vi "ENUM_Parse.vi"(8 "error":errorcluster, 9 "Secondary seporator(,)":string=",", 10 "Primary seperator(;)":string=";", 11 "Enum":variant) -> (0 "error out":errorcluster, 1 "Post Seperator array":string[](array[string]), 3 "Post Seperator":string, 5 "Name":string)   [LabVIEW 2015]
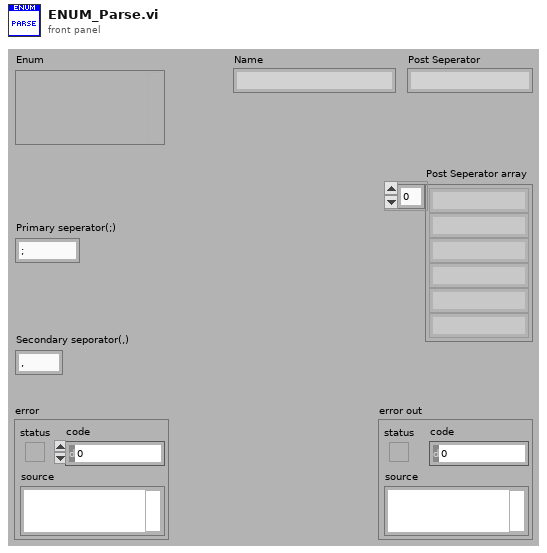
[diagram p1: front panel]
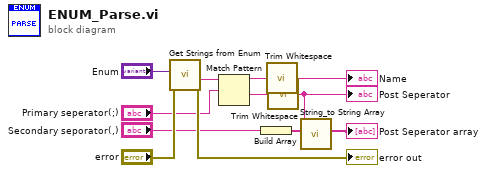
[diagram p0: block diagram]
diagram:
  n1 = call "Get Strings from Enum.vi"("error in (no error)"="error", "Enum"="Enum") -> ("error out"=→"error out":errorcluster, "String Value"=w1:string)  [unwired: 6 in, 2 out]
  n2 = Match Pattern(string=w1, regular expression="Primary seperator(;)") -> (before substring=w8:string, after substring=w6:string)  [unwired: 1 in, 2 out]
  n3 = Build Array("Secondary seporator(,)") -> (w3:string[])
  n4 = call <vilib>:"Trim Whitespace.vi"("string"=w8) -> ("trimmed string"=→"Name":string)  [unwired: 1 in]
  n5 = call <vilib>:"Trim Whitespace.vi"("string"=w6) -> ("trimmed string"=w5:string)  [unwired: 1 in]
  "Post Seperator" <- w5
  n6 = call "String_to String Array.vi"("Seperators (;)"=w3, "Input String"=w5) -> ("String Array Out Blanks Removed Out"=→"Post Seperator array":string[])  [unwired: 7 in, 2 out]
